vi "FlushTxRx.vi"(10 "error in (no error)":errorcluster, 11 "FPGA VI Reference In":T1) -> (2 "error out":errorcluster, 3 "FPGA VI Reference Out":T1)   [LabVIEW 2016]
uses:
  FPGA Bitfiles/FPGA_defref.ctl
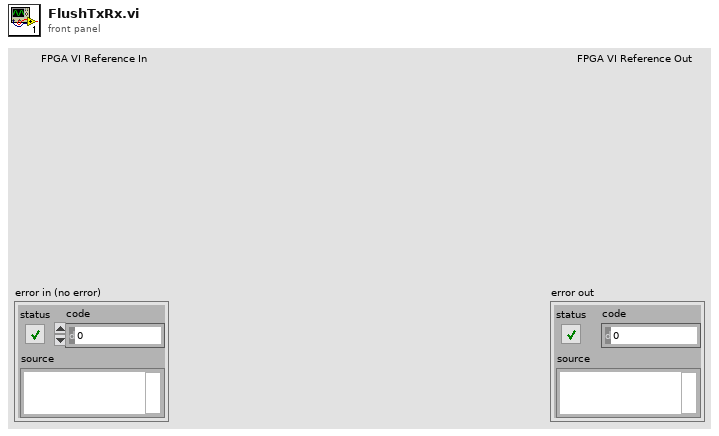
[diagram p1: front panel]
types:
  T1 = typedef "FPGA_defref.ctl" = refnum<k20>
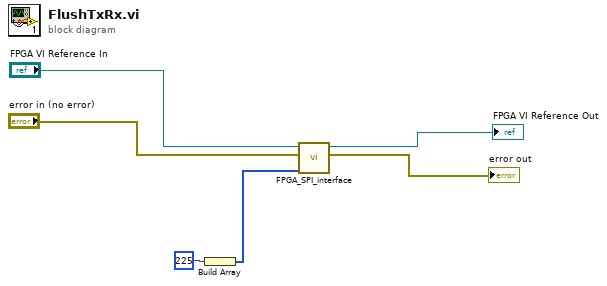
[diagram p0: block diagram]
diagram:
  n1 = Build Array(225) -> (w3:i32[])
  n2 = call "FPGA_SPI_interface.vi"("Frames to Write"=w3, "error in"="error in (no error)", "FPGA VI Reference In"="FPGA VI Reference In") -> ("error out"=→"error out":errorcluster, "FPGA VI Reference Out"=→"FPGA VI Reference Out":T1)  [unwired: 6 in, 1 out]
